vi "State Dequeue.vi"(8 "error in (no error)":errorcluster, 11 "Control Ref Queue":T2) -> (0 "error out":errorcluster, 1 "Action":T1)   [LabVIEW 2017, in "3D Plot.lvclass"]
uses:
  <vilib>/Math Plots/3D Math Plots/3D Plot/3D Plot/3D Plot.lvclass
  <vilib>/Math Plots/3D Math Plots/3D Plot/Action String/3DMathPlot Ctrl Act Queue.ctl
  <vilib>/Math Plots/3D Math Plots/3D Plot/Action String/3DMathPlot Ctrl Act Cluster.ctl
  <vilib>/Math Plots/3D Math Plots/3D Plot/Action String/3DMathPlot State Class.ctl
  <vilib>/Math Plots/3D Math Plots/3D Plot/3D Plot/Typedef/Plot Action.ctl
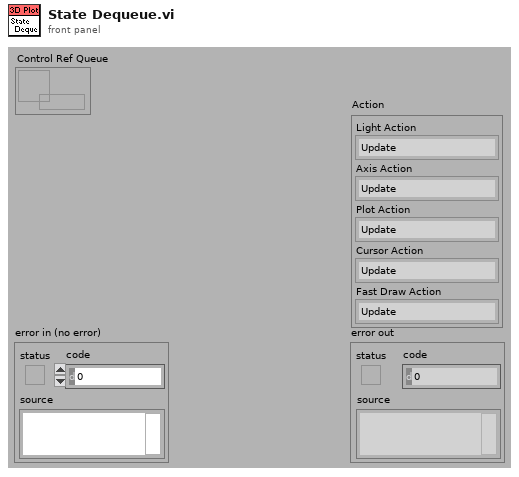
[diagram p1: front panel]
types:
  T1 = typedef "3D Plot.lvclass/Plot Action.ctl" = cluster{"Light Action":enum16{"Update", "Remove", "Nothing"}, "Axis Action":enum16{"Update", "Remove", "Nothing"}, "Plot Action":enum16{"Update", "Remove", "Nothing"}, "Cursor Action":enum16{"Update", "Remove", "Nothing"}, "Fast Draw Action":enum16{"Update", "Remove", "Nothing"}}
  T2 = typedef "3DMathPlot Ctrl Act Queue.ctl" = refnum<queue>
  T3 = typedef "3DMathPlot State Class.ctl" = enum16{"Update All Objects (Undo)", "Update Light Object Only", "Update Axis Object Only", "Update Plot Object Only", "Update Cursor Object Only", "Update Axis Plot Cursor Objects", "No Update"}
  T4 = typedef "3DMathPlot Ctrl Act Cluster.ctl" = cluster{"3D Picture Control":refnum<vi>, "Render Window Refnum":refnum<vi>, "XY Graph":refnum<vi>, "Intensity Graph":refnum<vi>, "Color Legend Palette":refnum<vi>, "Projection Palette":refnum<vi>, "XControl  Ref":refnum<vi>, "Facade Ref":refnum<vi>, "Export Image Ref":refnum<vi>, "Clear Data Flag":bool, "Display State Change Class":T3}
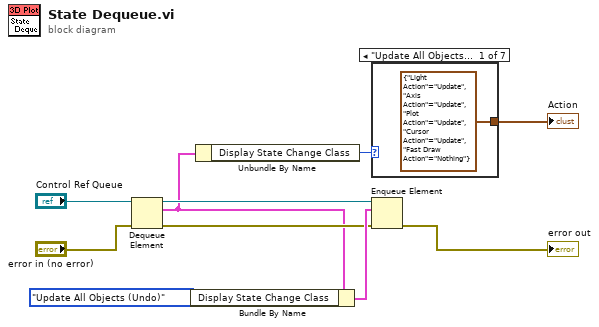
[diagram p0: block diagram]
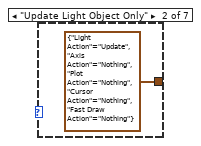
[diagram p2: hidden frame]
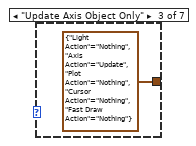
[diagram p3: hidden frame]
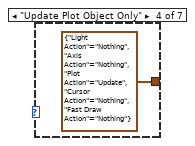
[diagram p4: hidden frame]
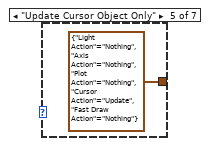
[diagram p5: hidden frame]
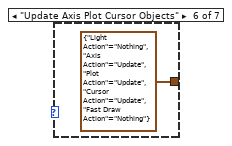
[diagram p6: hidden frame]
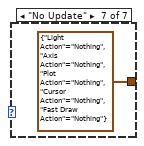
[diagram p7: hidden frame]
diagram:
  n1 = Dequeue Element(queue="Control Ref Queue", error in (no error)="error in (no error)") -> (queue out=w9:T2, element=w4:T4, error out=w7:errorcluster)  [unwired: 2 out]
  n2 = Bundle By Name(cluster=w4, "Display State Change Class"=3DMathPlot_State_Class."Update All Objects (Undo)") -> (w8:T4)
  n3 = Unbundle By Name(w4) -> ("Display State Change Class"=w1:T3)
  n4 = case shown="\"Update All Objects (Undo)\", Default" w1 {
    tunnel: [T1 {"Light Action"=enum."Update", "Axis Action"=enum."Update", "Plot Action"=enum."Update", "Cursor Action"=enum."Update", "Fast Draw Action"=enum."Nothing"} ("Action") T1 {"Light Action"=enum."Update", "Axis Action"=enum."Nothing", "Plot Action"=enum."Nothing", "Cursor Action"=enum."Nothing", "Fast Draw Action"=enum."Nothing"} ("Action") T1 {"Light Action"=enum."Nothing", "Axis Action"=enum."Update", "Plot Action"=enum."Nothing", "Cursor Action"=enum."Nothing", "Fast Draw Action"=enum."Nothing"} ("Action") T1 {"Light Action"=enum."Nothing", "Axis Action"=enum."Nothing", "Plot Action"=enum."Update", "Cursor Action"=enum."Nothing", "Fast Draw Action"=enum."Nothing"} ("Action") T1 {"Light Action"=enum."Nothing", "Axis Action"=enum."Nothing", "Plot Action"=enum."Nothing", "Cursor Action"=enum."Update", "Fast Draw Action"=enum."Nothing"} ("Action") T1 {"Light Action"=enum."Nothing", "Axis Action"=enum."Update", "Plot Action"=enum."Update", "Cursor Action"=enum."Update", "Fast Draw Action"=enum."Nothing"} ("Action") T1 {"Light Action"=enum."Nothing", "Axis Action"=enum."Nothing", "Plot Action"=enum."Nothing", "Cursor Action"=enum."Nothing", "Fast Draw Action"=enum."Nothing"} ("Action")] -> w2
    frame "Update All Objects (Undo)", Default {
    }
    frame "Update Light Object Only" {
    }
    frame "Update Axis Object Only" {
    }
    frame "Update Plot Object Only" {
    }
    frame "Update Cursor Object Only" {
    }
    frame "Update Axis Plot Cursor Objects" {
    }
    frame "No Update" {
    }
  }
  "Action" <- w2
  n5 = Enqueue Element(queue=w9, element=w8, error in (no error)=w7) -> (error out=→"error out":errorcluster)  [unwired: 3 out]
